vi "Send String.vi"(7 "Bus In":refnum<class "Bus.lvclass">, 8 "error in (no error)":errorcluster, 9 "Data Values":dbl[](array[numeric]), 10 "Data String":string, 11 "Parser in":refnum<class "Output.lvclass">) -> (0 "error out":errorcluster, 2 "Bus Out":refnum<class "Bus.lvclass">, 3 "Parser out":refnum<class "Output.lvclass">)   [LabVIEW 2018, in "Output.lvclass"]
doc: "Parserl.lvclass:Parse.vi\n\nThis is the template for the Parse VI for the Parser class.\n\nInstrument Communication Module Version 1.0\nSeptember, 2017 Original Code Consulting David Thomson\n www.originalcode.com"
uses:
  Output.lvclass
  Bus/Bus.lvclass
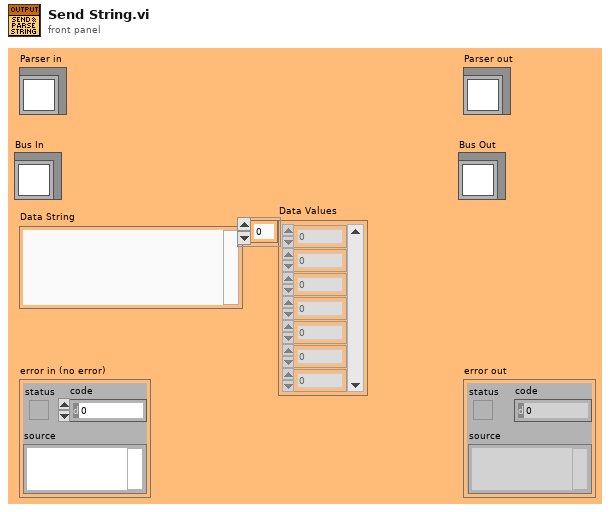
[diagram p1: front panel]
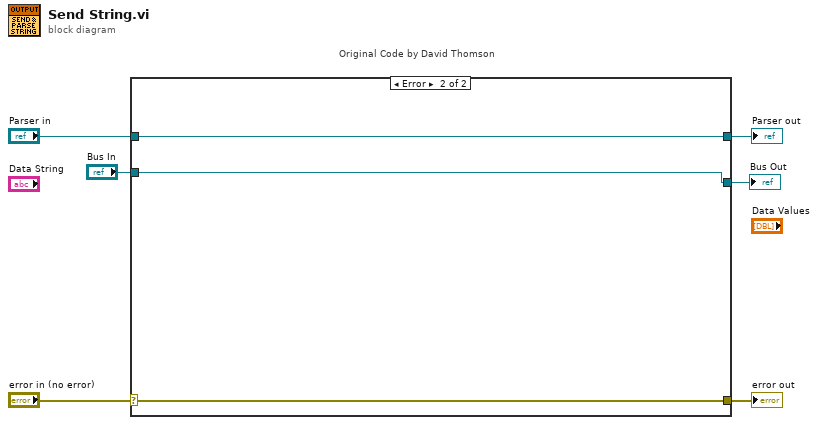
[diagram p0: block diagram]
diagram:
  n1 = case "Original Code by David Thomson" shown="Error" "error in (no error)" {
    selector: "error in (no error)" -> [w8 w12]
    tunnel: [w8 w12] -> w5
    tunnel: [w9 w11] -> w3
    tunnel: "Parser in" -> [w9 w11]
    tunnel: "Bus In" -> [w7 w10]
    tunnel: [w7 w10] -> w1
    frame No Error {
    }
    frame Error {
    }
  }
  "error out" <- w5
  "Parser out" <- w3
  "Bus Out" <- w1
